vi "test1dArrayTo2dArray.vi"(8 "error in (no error)":errorcluster) -> (0 "error out":errorcluster)   [LabVIEW 2016]
doc: "Test to transform the 1D array to 2D array."
uses:
  <vilib>/addons/_JKI Toolkits/Caraya/classes/Assert/Assert.lvclass
  <vilib>/addons/_JKI Toolkits/Caraya/classes/Test/Test.lvclass
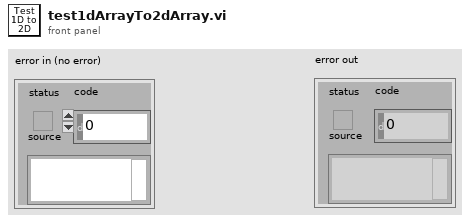
[diagram p1: front panel]
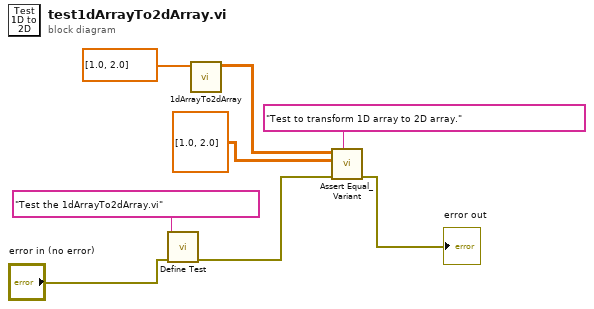
[diagram p0: block diagram]
diagram:
  n1 = call <vilib>:"Define Test.vi"("error in (no error)"="error in (no error)", "Label (VI Title)"="Test the 1dArrayTo2dArray.vi") -> ("error out"=w3:errorcluster)  [unwired: 9 in]
  n2 = call "1dArrayTo2dArray.vi"("1D Array"=dbl[] [1.0, 2.0]) -> ("2D Array"=w7:dbl[][])  [unwired: 10 in]
  n3 = call <vilib>:"Assert Equal_Variant.vi"("Label"="Test to transform 1D array to 2D array.", "error in (no error)"=w3, "Y"=dbl[][] [[1.0], [2.0]], "X"=w7) -> ("error out"=→"error out":errorcluster)  [unwired: 7 in]
